vi "PopUp Menu Item Manager.vi"() -> ()   [LabVIEW 2018]
uses:
  Support/File Collision Options.ctl
panel:
  in  "Help Button":bool
  out "Currently Running Version":string
  in  "Mass Compile":bool
  in  "Install for":u16(ring) items=["All Versions"]
  in  "Restart":bool
  in  "Uninstall":bool
  in  "Open Installed Folder":bool
  in  "Open Avail Folder":bool
  in  "Refresh":bool
  in  "Select New":bool
  in  "Select All Avail":bool
  in  "Close":bool
  in  "Install":bool
  in  "Items Installed":i32[](listbox) caption="Items Already Installed in\nC:\\Users\\BDTest\\Documents\\LabVIEW Data\\PopupMenus\\edit time panel and diagram"
  in  "Items Available":i32[](listbox) caption="Items Available in\nX:\\PERFORCE\\Source\\LabVIEW\\Common\\Utility\\Tools\\PopUp Menus"
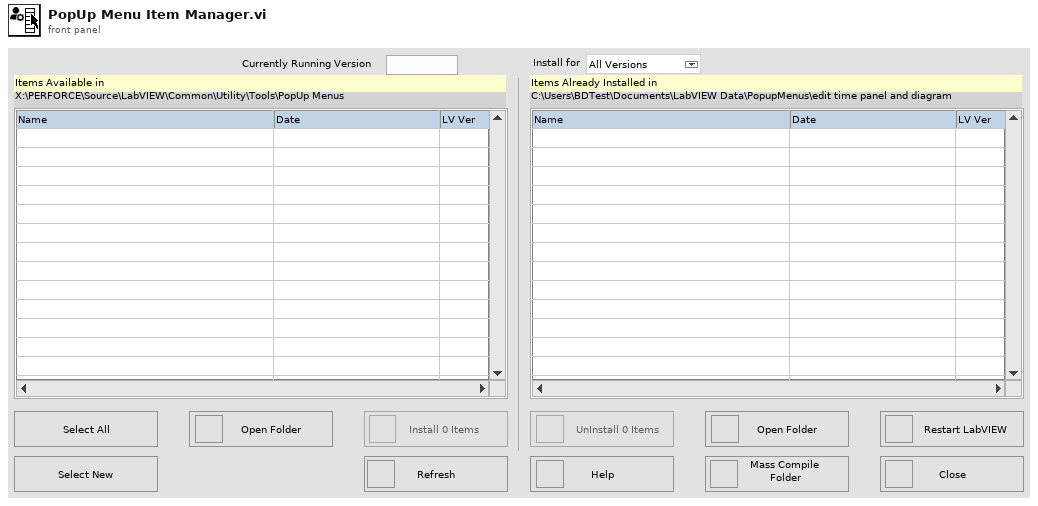
[diagram p1: front panel]
types:
  T1 = cluster{"Folder":path, "Item Paths":path[], "Descriptions":string[], "Names":string[], "TimeStamps":timestamp[]}
  T2 = enum8{"Enabled", "Disabled", "Disabled and Grayed Out"}
  T3 = typedef "File Collision Options.ctl" = cluster{"Dest is Newer & RO":enum16{"Throw Error", "Ask", "Skip", "Overwrite Siliently"}, "Dest is Newer & RW":enum16{"Throw Error", "Ask", "Skip", "Overwrite Siliently"}, "Dest is Older & RO":enum16{"Throw Error", "Ask", "Skip", "Overwrite Siliently"}, "Dest is Older & RW":enum16{"Throw Error", "Ask", "Skip", "Overwrite Siliently"}}
  T4 = cluster{"Name":string, "Description":string, "TimeStamp":timestamp, "LV Version":string, "Help Tag":string}
  T5 = typedef "LVPoint32TypeDef.ctl" = cluster{"Horizontal":i32, "Vertical":i32}
  T6 = typedef "LVRowAndColumnTypeDef.ctl" = cluster{"Row":i32, "Column":i32}
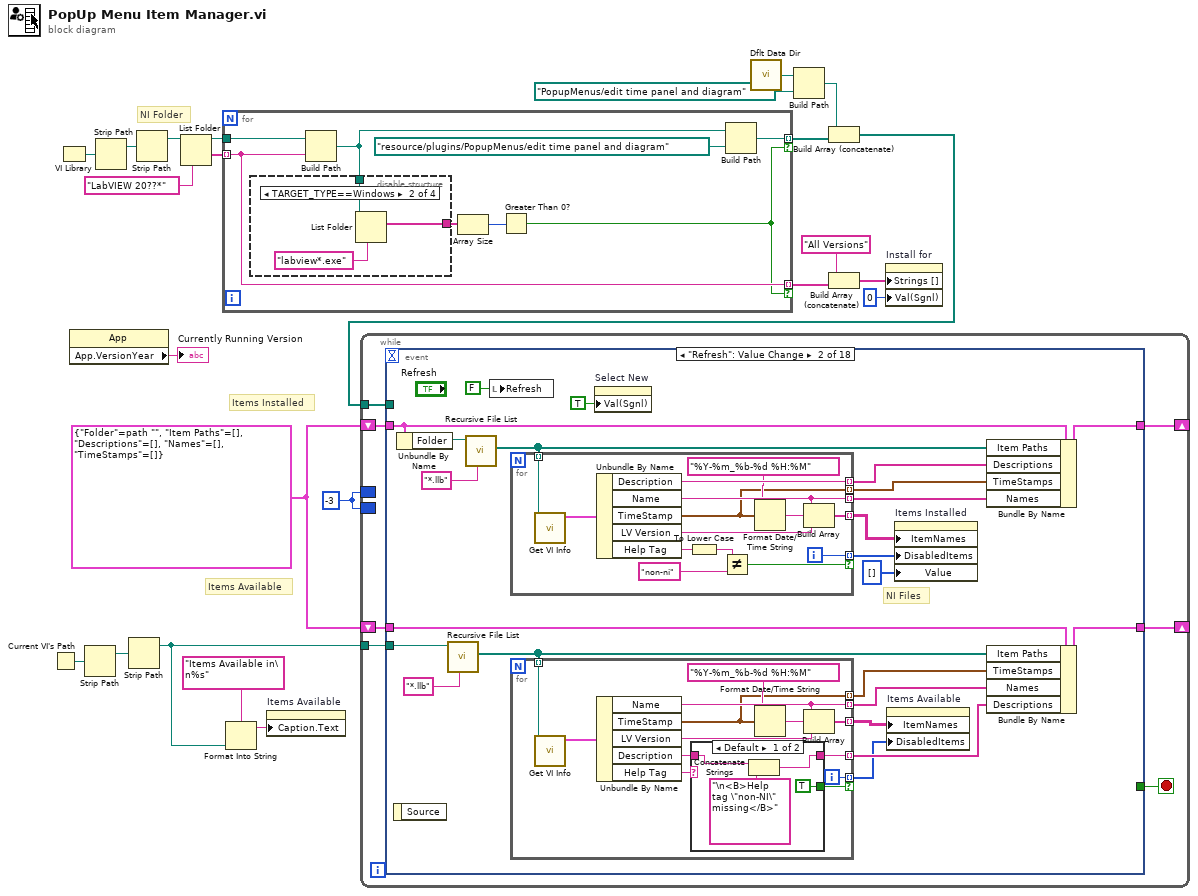
[diagram p0: block diagram]
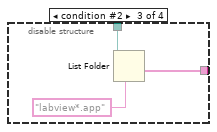
[diagram p3: hidden frame]
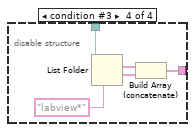
[diagram p4: hidden frame]
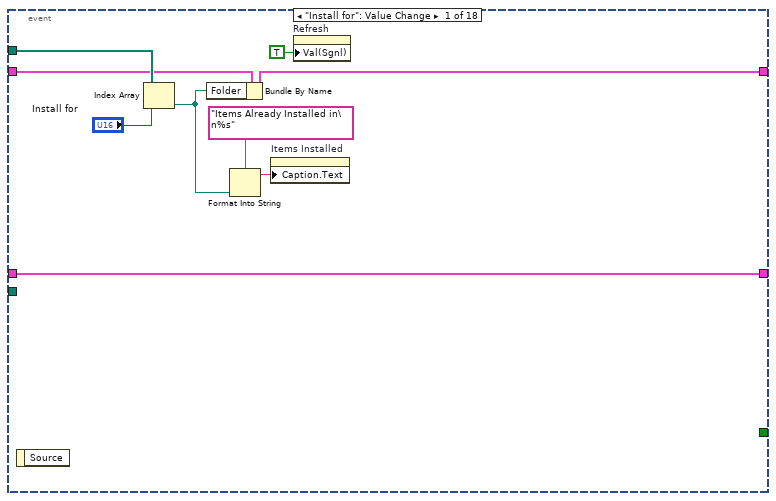
[diagram p5: hidden frame]
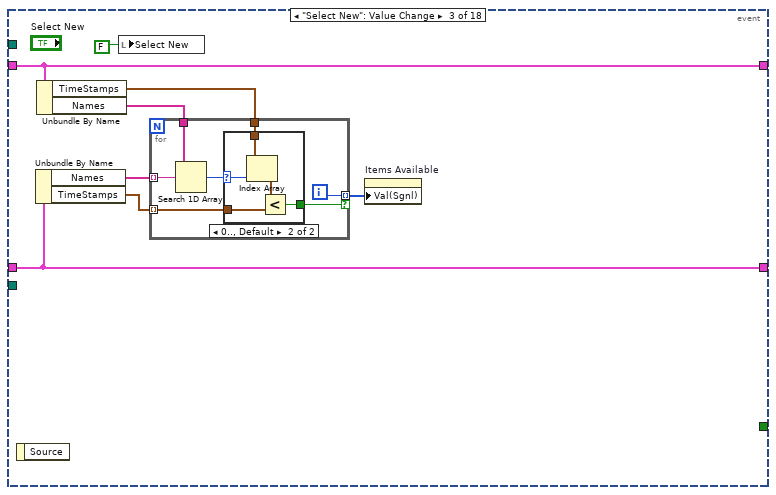
[diagram p7: hidden frame]
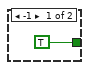
[diagram p8: hidden frame]
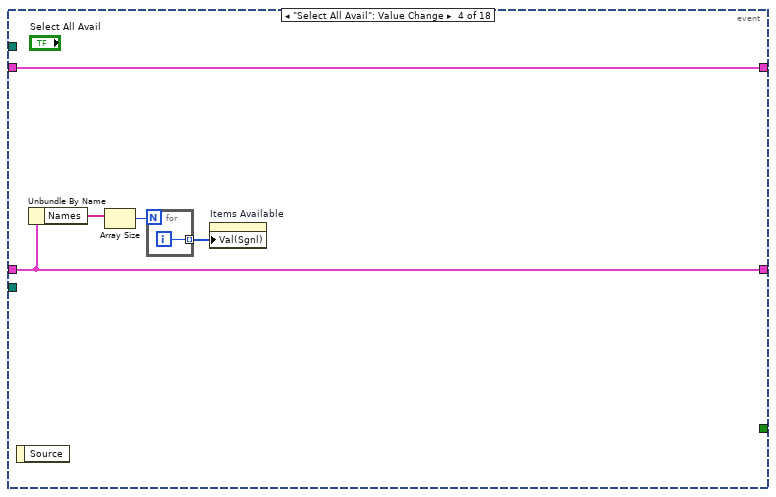
[diagram p9: hidden frame]
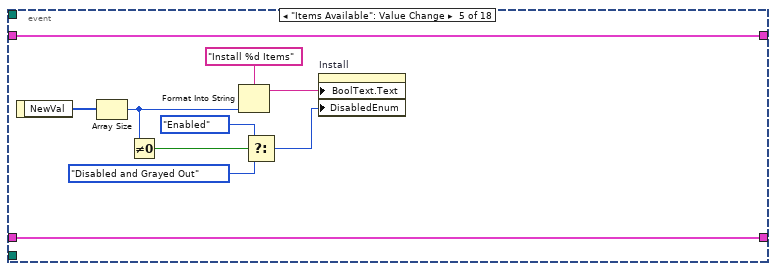
[diagram p10: hidden frame]
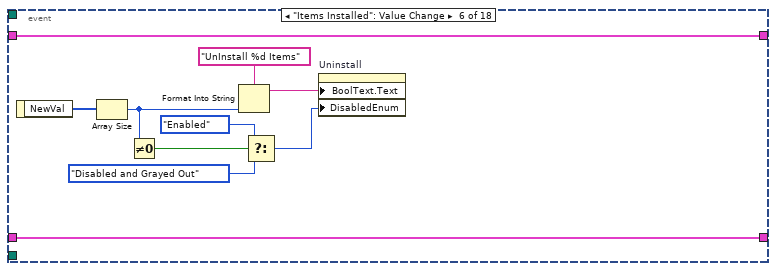
[diagram p11: hidden frame]
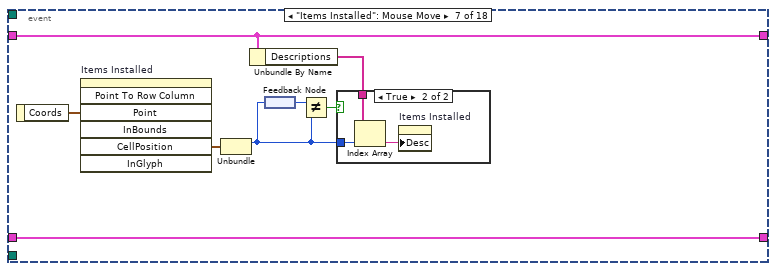
[diagram p12: hidden frame]
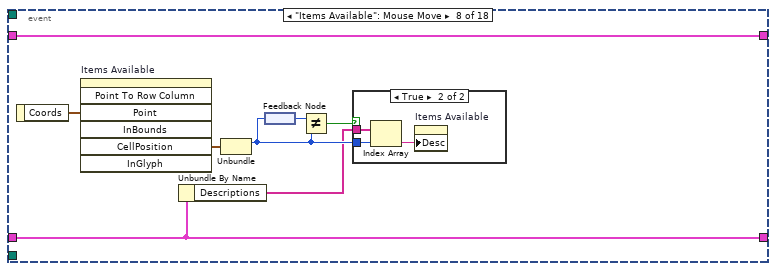
[diagram p14: hidden frame]
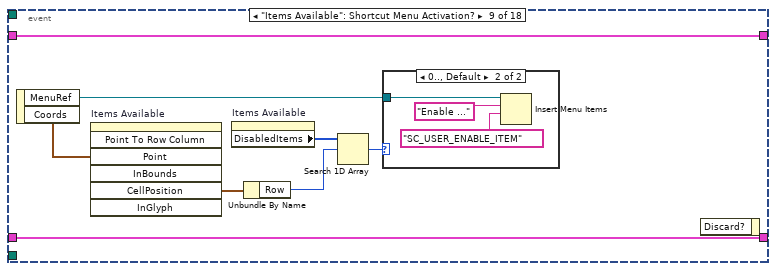
[diagram p16: hidden frame]
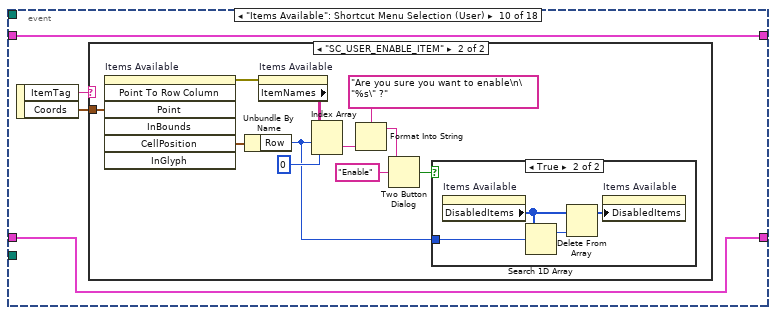
[diagram p18: hidden frame]
diagram:
  w6 = T1 {"Folder"=path "", "Item Paths"=[], "Descriptions"=[], "Names"=[], "TimeStamps"=[]}
  w5 = -3 ("Row")
  # "Items Available"
  # "Items Installed"
  # "NI Folder"
  n1 = Current VI's Path() -> (path=w1:path)
  n2 = VI Library() -> (path=w3:path)
  n3 = property on="Property Node" class="App"() -> ("App.VersionYear"=→"Currently Running Version":string)  [unwired: 2 in, 2 out]
  n4 = Strip Path(path=w1) -> (stripped path=w2:path)  [unwired: 1 out]
  n5 = Strip Path(path=w3) -> (stripped path=w20:path)  [unwired: 1 out]
  n6 = Strip Path(path=w2) -> (stripped path=w23:path)  [unwired: 1 out]
  n7 = Strip Path(path=w20) -> (stripped path=w16:path)  [unwired: 1 out]
  n8 = List Folder(path=w16, pattern="LabVIEW 20??*") -> (path out=w18:path, folder names=w17:string[])  [unwired: 2 in, 2 out]
  n9 = for {
    tunnel: w18 -> [w31]
    tunnel: w17 -> [w30] mode=indexing
    tunnel: [w28] -> w13 mode=indexing if=w26
    tunnel: [w30] -> w11 mode=indexing if=w26
    n10 = Build Path(base path=w31, name or relative path=w30) -> (appended path=w24:path)
    n11 = disable-structure shown="TARGET_TYPE==Windows" {
      disable-tunnel: [_ w33 w36 w39] -> w25
      disable-tunnel: w24 -> [_ w32 w35 w38]
      frame condition #0 {
      }
      frame condition #1 (active) {
        n12 = List Folder(path=w32, pattern="labview*.exe" ("name or relative path")) -> (filenames=w33:string[])  [unwired: 2 in, 3 out]
      }
      frame condition #2 {
        n13 = List Folder(path=w35, pattern="labview*.app" ("name or relative path")) -> (folder names=w36:string[])  [unwired: 2 in, 3 out]
      }
      frame condition #3 {
        n14 = List Folder(path=w38, pattern="labview*" ("name or relative path")) -> (filenames=w41:string[], folder names=w40:string[])  [unwired: 2 in, 2 out]
        n15 = Build Array (concatenate)(w41, w40) -> (w39:string[])
      }
    }
    n16 = Array Size(array=w25) -> (size(s)=w27:i32)
    n17 = Greater Than 0?(x=w27) -> (x > 0?=w26:bool)
    n18 = Build Path(base path=w24, name or relative path=path "resource/plugins/PopupMenus/edit time panel and diagram") -> (appended path=w28:path)
  }
  n19 = Format Into String(format string="Items Available in\n%s", w23) -> (resulting string=w21:string)  [unwired: 2 in, 1 out]
  n20 = property on="Items Available" class="MCListbox (strict)"("Caption.Text"=w21) -> ()  [unwired: 2 in, 2 out]
  n21 = call <vilib>:"Dflt Data Dir.vi"() -> ("App:Default Data Directory"=w15:path)
  n22 = Build Path(base path=w15, name or relative path=path "PopupMenus/edit time panel and diagram") -> (appended path=w12:path)
  n23 = Build Array (concatenate)(w12, w13) -> (w8:path[])
  n24 = while {
    tunnel: w23 -> [w48]
    border: w5 -> [_]
    border: w5 -> [_]
    shift-right: [w45] -> _
    shift-left: w6 -> [w47]
    tunnel: w8 -> [w46]
    shift-right: [w43] -> _
    shift-left: w6 -> [w44]
    stop <- w49 stop-if-true
    n25 = event shown="[1] \"Refresh\": Value Change" {
      selector: _ -> [_ _ _ _ _ _ _ _ _ _ _ _ _ _ _ _ _ _]
      dyn-events: _ -> [_ _ _ _ _ _ _ _ _ _ _ _ _ _ _ _ _ _]
      timeout: _ -> [_ _ _ _ _ _ _ _ _ _ _ _ _ _ _ _ _ _]
      tunnel: [_ _ _ _ _ _ _ _ _ _ _ _ _ _ _ _ "Close" "Restart"] -> w49
      tunnel: w48 -> [_ w76 _ _ _ _ _ _ _ _ _ _ w243 _ _ _ _ _]
      tunnel: w47 -> [w56 w72 w119 w137 w144 w160 w162 w174 w190 w197 w217 w229 w247 w251 w259 w273 w275 w281]
      tunnel: w46 -> [w58 _ _ _ _ _ _ _ _ _ _ _ _ _ _ _ _ _]
      tunnel: [w55 w75 w119 w137 w144 w160 w162 w174 w190 w197 w217 w229 w247 w251 w259 w273 w275 w281] -> w45
      tunnel: w44 -> [w50 w74 w117 w136 w143 w159 w163 w173 w189 w194 w215 w230 w246 w252 w260 w272 w274 w280]
      tunnel: [w50 w73 w117 w136 w143 w159 w163 w173 w189 w194 w215 w230 w246 w252 w260 w272 w274 w280] -> w43
      event "Install for": Value Change {
        n26 = event-data() -> ()  [unwired: 1 in, 1 out]
        n27 = Index Array(array=w58, index="Install for") -> (element=w51:path)
        n28 = Bundle By Name(cluster=w56, "Folder"=w51) -> (w55:T1)
        n29 = Format Into String(format string="Items Already Installed in\n%s", w51) -> (resulting string=w52:string)  [unwired: 2 in, 1 out]
        n30 = property on="Items Installed" class="MCListbox (strict)"("Caption.Text"=w52) -> ()  [unwired: 2 in, 2 out]
        n31 = property on="Refresh" class="Bool (strict)"("Val(Sgnl)"=TRUE ("Value (Signaling)")) -> ()  [unwired: 2 in, 2 out]
      }
      event "Refresh": Value Change {
        # "NI Files"
        n32 = event-data() -> ()  [unwired: 1 in, 1 out]
        n33 = Unbundle By Name(w72) -> ("Folder"=w71:path)
        n34 = call <vilib>:"Recursive File List.vi"("pattern"="*.llb", "Folder Path"=w76) -> ("All Files in Dir"=w61:path[])  [unwired: 5 in, 4 out]
        n35 = call <vilib>:"Recursive File List.vi"("pattern"="*.llb", "Folder Path"=w71) -> ("All Files in Dir"=w70:path[])  [unwired: 5 in, 4 out]
        n36 = local write "Refresh"(FALSE ("Refresh")) -> ()
        n37 = for {
          tunnel: w70 -> [w113] mode=indexing
          tunnel: [w111] -> w68 mode=indexing
          tunnel: [w106] -> w69 mode=indexing
          tunnel: [w110] -> w67 mode=indexing
          tunnel: [w109] -> w66 mode=indexing if=w101
          tunnel: [w104] -> w65 mode=indexing
          i -> [w109]
          n38 = call "Get VI Info.vi"("VI Path"=w113) -> ("VI Info"=w112:T4)  [unwired: 7 in, 1 out]
          n39 = Unbundle By Name(w112) -> ("Description"=w106:string, "Name"=w111:string, "TimeStamp"=w104:timestamp, "LV Version"=w108:string, "Help Tag"=w103:string)
          n40 = To Lower Case(string=w103) -> (all lower case string=w100:string)
          n41 = Not Equal?(x=w100, y="non-ni") -> (x != y?=w101:bool)
          n42 = Format Date/Time String(time format string (%c)="%Y-%m_%b-%d %H:%M" ("TimeStamp Format"), seconds (now)=w104) -> (date/time string=w107:string)  [unwired: 1 in]
          n43 = Build Array(w111, w107, w108) -> (w110:string[])
        }
        n44 = for {
          tunnel: w61 -> [w94] mode=indexing
          tunnel: [w92] -> w63 mode=indexing
          tunnel: [w84] -> w60 mode=indexing
          tunnel: [w91] -> w62 mode=indexing
          tunnel: [w87] -> w64 mode=indexing
          tunnel: [w83] -> w59 mode=indexing if=w82
          i -> [w83]
          n45 = call "Get VI Info.vi"("VI Path"=w94) -> ("VI Info"=w93:T4)  [unwired: 7 in, 1 out]
          n46 = Unbundle By Name(w93) -> ("Name"=w92:string, "TimeStamp"=w87:timestamp, "LV Version"=w90:string, "Description"=w85:string, "Help Tag"=w86:string)
          n47 = case shown="Default" w86 {
            tunnel: w85 -> [w97 w99]
            tunnel: [w96 w99] -> w84
            tunnel: [TRUE _] -> w82
            frame Default {
              n48 = Concatenate Strings(w97, "\n<B>Help tag \"non-NI\" missing</B>" ("string")) -> (w96:string)
            }
            frame "non-NI" {
            }
          }
          n49 = Format Date/Time String(time format string (%c)="%Y-%m_%b-%d %H:%M" ("TimeStamp Format"), seconds (now)=w87) -> (date/time string=w89:string)  [unwired: 1 in]
          n50 = Build Array(w92, w89, w90) -> (w91:string[])
        }
        n51 = property on="Select New" class="Bool (strict)"("Val(Sgnl)"=TRUE ("Value (Signaling)")) -> ()  [unwired: 2 in, 2 out]
        n52 = property on="Items Available" class="MCListbox (strict)"("ItemNames"=w62, "DisabledItems"=w59) -> ()  [unwired: 2 in, 2 out]
        n53 = property on="Items Installed" class="MCListbox (strict)"("ItemNames"=w67, "DisabledItems"=w66, "Value"=i32[] [] ("Items Installed")) -> ()  [unwired: 2 in, 2 out]
        n54 = Bundle By Name(cluster=w72, "Item Paths"=w70, "Descriptions"=w69, "TimeStamps"=w65, "Names"=w68) -> (w75:T1)
        n55 = Bundle By Name(cluster=w74, "Item Paths"=w61, "TimeStamps"=w64, "Names"=w63, "Descriptions"=w60) -> (w73:T1)
      }
      event "Select New": Value Change {
        n56 = event-data() -> ()  [unwired: 1 in, 1 out]
        n57 = Unbundle By Name(w117) -> ("Names"=w116:string[], "TimeStamps"=w115:timestamp[])
        n58 = Unbundle By Name(w119) -> ("TimeStamps"=w118:timestamp[], "Names"=w114:string[])
        n59 = local write "Select New"(FALSE ("Select New")) -> ()
        n60 = for {
          tunnel: w116 -> [w127] mode=indexing
          tunnel: w114 -> [w128]
          tunnel: [w125] -> w121 mode=indexing if=w124
          tunnel: w115 -> [w123] mode=indexing
          tunnel: w118 -> [w122]
          i -> [w125]
          n61 = Search 1D Array(1D array=w128, element=w127) -> (index of element=w126:i32)  [unwired: 1 in]
          n62 = case shown="0.., Default" w126 {
            selector: w126 -> [_ w134]
            tunnel: [TRUE w132] -> w124
            tunnel: w123 -> [_ w131]
            tunnel: w122 -> [_ w130]
            frame -1 {
            }
            frame 0.., Default {
              n63 = Index Array(array=w130, index=w134) -> (element=w133:timestamp)
              n64 = Less?(x=w133, y=w131) -> (x < y?=w132:bool)
            }
          }
        }
        n65 = property on="Items Available" class="MCListbox (strict)"("Val(Sgnl)"=w121) -> ()  [unwired: 2 in, 2 out]
      }
      event "Select All Avail": Value Change {
        n66 = event-data() -> ()  [unwired: 1 in, 1 out]
        n67 = Unbundle By Name(w136) -> ("Names"=w135:string[])
        n68 = Array Size(array=w135) -> (size(s)=w139:i32)
        n69 = for {
          N: w139 -> [_]
          tunnel: [w140] -> w138 mode=indexing
          i -> [w140]
        }
        n70 = property on="Items Available" class="MCListbox (strict)"("Val(Sgnl)"=w138) -> ()  [unwired: 2 in, 2 out]
      }
      event "Items Available": Value Change {
        n71 = event-data() -> ("NewVal"=w145:i32[])  [unwired: 1 in]
        n72 = Array Size(array=w145) -> (size(s)=w148:i32)
        n73 = Not Equal To 0?(x=w148) -> (x != 0?=w147:bool)
        n74 = Format Into String(format string="Install %d Items", w148) -> (resulting string=w149:string)  [unwired: 2 in, 1 out]
        n75 = Select(t=T2."Enabled" ("Disabled"), s=w147, f=T2."Disabled and Grayed Out" ("Disabled")) -> (s? t:f=w146:T2)
        n76 = property on="Install" class="Bool"("BoolText.Text"=w149, "DisabledEnum"=w146) -> ()  [unwired: 2 in, 2 out]
      }
      event "Items Installed": Value Change {
        n77 = event-data() -> ("NewVal"=w151:i32[])  [unwired: 1 in]
        n78 = Array Size(array=w151) -> (size(s)=w156:i32)
        n79 = Not Equal To 0?(x=w156) -> (x != 0?=w155:bool)
        n80 = Format Into String(format string="UnInstall %d Items", w156) -> (resulting string=w157:string)  [unwired: 2 in, 1 out]
        n81 = Select(t=T2."Enabled" ("Disabled"), s=w155, f=T2."Disabled and Grayed Out" ("Disabled")) -> (s? t:f=w154:T2)
        n82 = property on="Uninstall" class="Bool"("BoolText.Text"=w157, "DisabledEnum"=w154) -> ()  [unwired: 2 in, 2 out]
      }
      event "Items Installed": Mouse Move {
        n83 = event-data() -> ("Coords"=w168:T5)  [unwired: 1 in]
        n84 = invoke on="Items Installed" class="MCListbox (strict)" method="Point To Row Column"("Point"=w168) -> ("CellPosition"=w167:T6)  [unwired: 6 in, 6 out]
        n85 = Unbundle(w167) -> ("Row"=w166:i32)  [unwired: 1 out]
        n86 = Unbundle By Name(w162) -> ("Descriptions"=w161:string[])
        n87 = feedback-in #1(w166) -> ()
        n88 = feedback #1() -> (w165:i32)
        n89 = Not Equal?(x=w165, y=w166) -> (x != y?=w164:bool)
        n90 = case shown="True" w164 {
          tunnel: w166 -> [_ w171]
          tunnel: w161 -> [_ w170]
          frame False {
          }
          frame True {
            n91 = Index Array(array=w170, index=w171) -> (element=w169:string)
            n92 = property on="Items Installed" class="MCListbox (strict)"("Desc"=w169) -> ()  [unwired: 2 in, 2 out]
          }
        }
      }
      event "Items Available": Mouse Move {
        n93 = event-data() -> ("Coords"=w179:T5)  [unwired: 1 in]
        n94 = invoke on="Items Available" class="MCListbox (strict)" method="Point To Row Column"("Point"=w179) -> ("CellPosition"=w178:T6)  [unwired: 6 in, 6 out]
        n95 = Unbundle By Name(w173) -> ("Descriptions"=w172:string[])
        n96 = Unbundle(w178) -> ("Row"=w175:i32)  [unwired: 1 out]
        n97 = feedback-in #2(w175) -> ()
        n98 = feedback #2() -> (w177:i32)
        n99 = Not Equal?(x=w177, y=w175) -> (x != y?=w176:bool)
        n100 = case shown="True" w176 {
          tunnel: w175 -> [_ w182]
          tunnel: w172 -> [_ w180]
          frame False {
          }
          frame True {
            n101 = Index Array(array=w180, index=w182) -> (element=w181:string)
            n102 = property on="Items Available" class="MCListbox (strict)"("Desc"=w181) -> ()  [unwired: 2 in, 2 out]
          }
        }
      }
      event "Items Available": Shortcut Menu Activation? {
        n103 = event-data() -> ("MenuRef"=w184:refnum<k9>, "Coords"=w183:T5)  [unwired: 1 in]
        n104 = invoke on="Items Available" class="MCListbox (strict)" method="Point To Row Column"("Point"=w183) -> ("CellPosition"=w188:T6)  [unwired: 6 in, 6 out]
        n105 = property on="Items Available" class="MCListbox (strict)"() -> ("DisabledItems"=w187:i32[])  [unwired: 2 in, 2 out]
        n106 = Unbundle By Name(w188) -> ("Row"=w186:i32)
        n107 = Search 1D Array(1D array=w187, element=w186) -> (index of element=w185:i32)  [unwired: 1 in]
        n108 = case shown="0.., Default" w185 {
          tunnel: w184 -> [_ w193]
          frame -1 {
          }
          frame 0.., Default {
            n109 = Insert Menu Items(7:"SC_USER_ENABLE_ITEM" ("item tags"), 8:"Enable ...", 9:w193) -> ()  [unwired: 3 in, 3 out]
          }
        }
        n110 = event-data() -> ()  [unwired: 2 in, 1 out]
      }
      event "Items Available": Shortcut Menu Selection (User) {
        n111 = event-data() -> ("ItemTag"=w196:string, "Coords"=w195:T5)  [unwired: 1 in]
        n112 = case shown="\"SC_USER_ENABLE_ITEM\"" w196 {
          tunnel: w195 -> [_ w208]
          frame Default {
          }
          frame "SC_USER_ENABLE_ITEM" {
            n113 = invoke on="Items Available" class="MCListbox (strict)" method="Point To Row Column"("Point"=w208) -> (error out=w206:errorcluster, "CellPosition"=w207:T6)  [unwired: 6 in, 5 out]
            n114 = Unbundle By Name(w207) -> ("Row"=w199:i32)
            n115 = property on="Items Available" class="MCListbox (strict)"(error in=w206) -> ("ItemNames"=w205:string[][])  [unwired: 1 in, 2 out]
            n116 = Index Array(array=w205, index (row)=w199, index (col)=0 ("disabled index (col)")) -> (element=w203:string)
            n117 = Format Into String(format string="Are you sure you want to enable\n\"%s\" ?", w203) -> (resulting string=w201:string)  [unwired: 2 in, 1 out]
            n118 = Two Button Dialog(message=w201, 2:"Enable" ("T button name (\"OK\")")) -> (T button?=w198:bool)  [unwired: 1 in]
            n119 = case shown="True" w198 {
              tunnel: w199 -> [_ w212]
              frame False {
              }
              frame True {
                n120 = property on="Items Available" class="MCListbox (strict)"() -> ("DisabledItems"=w210:i32[])  [unwired: 2 in, 2 out]
                n121 = Search 1D Array(1D array=w210, element=w212) -> (index of element=w211:i32)  [unwired: 1 in]
                n122 = Delete From Array(array=w210, index=w211) -> (array with subset deleted=w209:i32[])  [unwired: 1 in, 1 out]
                n123 = property on="Items Available" class="MCListbox (strict)"("DisabledItems"=w209) -> ()  [unwired: 2 in, 2 out]
              }
            }
          }
        }
      }
      event "Install": Value Change {
        n124 = event-data() -> ()  [unwired: 1 in, 1 out]
        n125 = Unbundle By Name(w215) -> ("Item Paths"=w214:path[])
        n126 = property on="Refresh" class="Bool (strict)"("Val(Sgnl)"=TRUE ("Value (Signaling)")) -> ()  [unwired: 2 in, 2 out]
        n127 = Unbundle By Name(w217) -> ("Folder"=w216:path)
        n128 = for {
          tunnel: w214 -> [w225]
          tunnel: w216 -> [w223]
          tunnel: "Items Available" -> [w226] mode=indexing
          border: FALSE ("Use same answer for all") -> [_]
          n129 = Index Array(array=w225, index=w226) -> (element=w224:path)
          n130 = feedback #3() -> (w221:bool)
          n131 = call "Copy File with Ask.vi"("Use Prev Answer"=w221, "On File Coillision"=T3 {"Dest is Newer & RO"=enum."Ask", "Dest is Newer & RW"=enum."Ask", "Dest is Older & RO"=enum."Ask", "Dest is Older & RW"=enum."Overwrite Siliently"}, "Destination Folder"=w223, "Source File"=w224) -> ("Use same answer for all"=w222:bool)  [unwired: 5 in, 2 out]
          n132 = feedback-in #3(w222) -> ()
        }
      }
      event "Uninstall": Value Change {
        n133 = event-data() -> ()  [unwired: 1 in, 1 out]
        n134 = Array Size(array="Items Installed") -> (size(s)=w235:i32)
        n135 = Format Into String(format string="Are you sure you want\nto delete %d files?", w235) -> (resulting string=w233:string)  [unwired: 2 in, 1 out]
        n136 = Two Button Dialog(message=w233, 2:"Delete" ("T button name (\"OK\")")) -> (T button?=w231:bool)  [unwired: 1 in]
        n137 = Unbundle By Name(w229) -> ("Item Paths"=w228:path[])
        n138 = case shown="True" w231 {
          tunnel: w228 -> [_ w239]
          tunnel: "Items Installed" -> [_ w238]
          frame False {
          }
          frame True {
            n139 = for {
              tunnel: w238 -> [w242] mode=indexing
              tunnel: w239 -> [w241]
              n140 = Index Array(array=w241, index=w242) -> (element=w240:path)
              n141 = Delete(path (use dialog)=w240) -> ()  [unwired: 4 in, 3 out]
            }
            n142 = property on="Refresh" class="Bool (strict)"("Val(Sgnl)"=TRUE ("Value (Signaling)")) -> ()  [unwired: 2 in, 2 out]
          }
        }
        n143 = property on="Uninstall" class="Bool"("BoolText.Text"="UnInstall 0 Items" ("format string")) -> ()  [unwired: 2 in, 2 out]
      }
      event "Open Avail Folder": Value Change {
        n144 = event-data() -> ()  [unwired: 1 in, 1 out]
        n145 = Format Into String(format string="Explorer \"%s\"", w243) -> (resulting string=w244:string)  [unwired: 2 in, 1 out]
        n146 = call <vilib>:"System Exec.vi"("command line"=w244) -> ()  [unwired: 7 in, 4 out]
      }
      event "Open Installed Folder": Value Change {
        n147 = event-data() -> ()  [unwired: 1 in, 1 out]
        n148 = Unbundle By Name(w251) -> ("Folder"=w250:path)
        n149 = Format Into String(format string="Explorer \"%s\"", w250) -> (resulting string=w248:string)  [unwired: 2 in, 1 out]
        n150 = call <vilib>:"System Exec.vi"("command line"=w248) -> ()  [unwired: 7 in, 4 out]
      }
      event "Mass Compile": Value Change {
        n151 = event-data() -> ()  [unwired: 1 in, 1 out]
        n152 = Unbundle By Name(w259) -> ("Folder"=w253:path)
        n153 = Format Into String(format string="Mass Compile\n%s", w253) -> (resulting string=w255:string)  [unwired: 2 in, 1 out]
        n154 = Two Button Dialog(message=w255, 1:"NO" ("F button name (\"Cancel\")"), 2:"YES" ("T button name (\"OK\")")) -> (T button?=w258:bool)
        n155 = case shown="True" w258 {
          tunnel: w253 -> [_ w261]
          frame False {
          }
          frame True {
            n156 = invoke class="App" method="Mass Compile"("Directory to Compile"=w261) -> ()  [unwired: 8 in, 9 out]
          }
        }
      }
      event "Help Button": Value Change {
        n157 = event-data() -> ()  [unwired: 1 in, 1 out]
        n158 = property on="Property Node" class="VI"() -> ("Path"=w268:path)  [unwired: 2 in, 2 out]
        n159 = Strip Path(path=w268) -> (stripped path=w266:path, name=w267:string)
        n160 = Build Path(base path=w266, name or relative path=path "Support" ("stripped path")) -> (appended path=w264:path)
        n161 = Search and Replace String(input string=w267, search string=".vi$", replace string=".chm" ("replace string (\"\")")) -> (result string=w263:string)  [unwired: 5 in, 3 out]
        n162 = Build Path(base path=w264, name or relative path=w263) -> (appended path=w262:path)
        n163 = Control Online Help(2:w262, 4:enum16{"Contents", "Key", "Close"}."Contents" ("Operation")) -> ()  [unwired: 2 in, 1 out]
      }
      event "Close": Value Change {
        n164 = event-data() -> ()  [unwired: 1 in, 1 out]
        n165 = disable-structure shown="Enabled" {
          frame Disabled {
            w279 = string[][] [] ("Item Names")
            n166 = property on="Items Available" class="MCListbox (strict)"("ItemNames"=w279) -> ()  [unwired: 2 in, 2 out]
            n167 = property on="Items Installed" class="MCListbox (strict)"("ItemNames"=w279) -> ()  [unwired: 2 in, 2 out]
            n168 = property on="Items Available" class="MCListbox (strict)"("Caption.Text"="Items Available in\n" ("format string")) -> ()  [unwired: 2 in, 2 out]
            n169 = property on="Items Installed" class="MCListbox (strict)"("Caption.Text"="Items Already Installed in\n" ("format string")) -> ()  [unwired: 2 in, 2 out]
          }
          frame Enabled {
            n170 = invoke class="VI" method="FP.Close"() -> ()  [unwired: 3 in, 3 out]
          }
        }
      }
      event "Restart": Value Change {
        n171 = event-data() -> ()  [unwired: 1 in, 1 out]
        n172 = invoke class="VI" method="FP.Close"() -> (error out=w282:errorcluster)  [unwired: 3 in, 2 out]
        n173 = invoke class="App" method="Restart"(error in=w282) -> ()  [unwired: 2 in, 3 out]
      }
    }
  }
  n174 = Build Array (concatenate)("All Versions" ("element"), w11) -> (w10:string[])
  n175 = property on="Install for" class="Ring (strict)"("Strings []"=w10, "Val(Sgnl)"=u16 0 ("Value (Signaling)")) -> ()  [unwired: 2 in, 2 out]
